vi "eventos.vi"() -> ()   [LabVIEW 2019]
uses:
  <vilib>/event_ctls.llb/eventvkey.ctl
panel:
  in  "MOUSE":bool
  out "ScanCode":i16
  out "PlatMods":T1
  out "VKey":T2
  out "Char":i16
  out "NewVal":bool
  out "OldVal":bool
  in  "Boolean":bool
  out "cuenta":i32
  in  "stop":bool
  in  "OK Button":bool
  out "iteraciones 1":i32
  out "LED 2":bool
  out "LED 1":bool
  # "EVENTO\nTECLADO"
  # "EVENTO\nCHANGE VALUE"
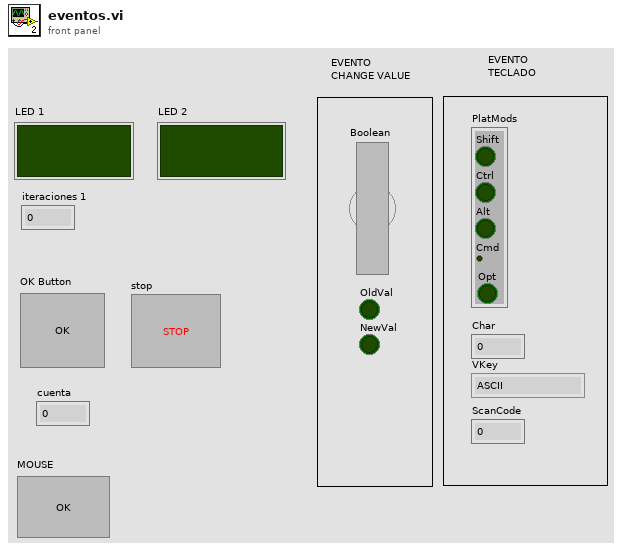
[diagram p1: front panel]
types:
  T1 = cluster{"Shift":bool, "Ctrl":bool, "Alt":bool, "Cmd":bool, "Opt":bool}
  T2 = typedef "eventvkey.ctl" = enum16{"ASCII", "Enter", "Return", "Shift", "Ctrl", "Alt", "Cmd", "Opt", "Caps", "NumLock", "Clear", "Break", "Up", "Down", "Left", "Right", "Insert", "Delete", "Home", "End", "PageUp", "PageDown", "Escape", "Help", "Pause", "ScrollLock", "F1", "F2", "F3", "F4", "F5", "F6", "F7", "F8", "F9", "F10", "F11", "F12", "F13", "F14", "F15", "F16", "F17", "F18", "F19", "F20", "F21", "F22", "F23", "F24", "Play", "VolumeUp", "VolumeDown", "Mute", "Two Byte Char"}
  T3 = typedef "LVPositionTypeDef.ctl" = cluster{"Left":i32, "Top":i32}
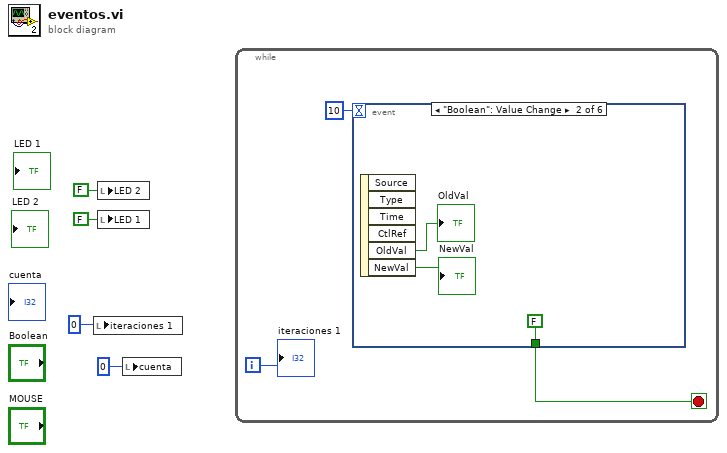
[diagram p0: block diagram]
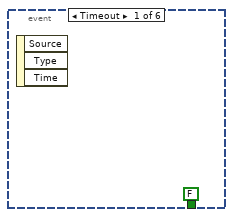
[diagram p2: hidden frame]
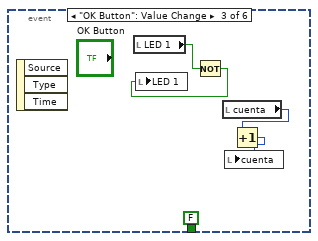
[diagram p3: hidden frame]
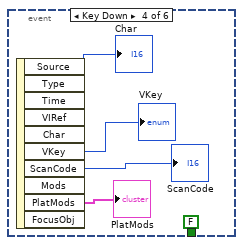
[diagram p4: hidden frame]
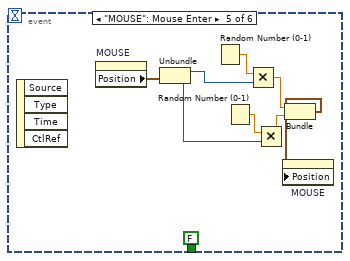
[diagram p5: hidden frame]
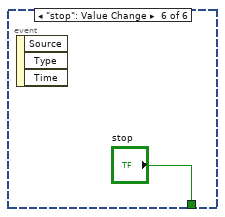
[diagram p6: hidden frame]
diagram:
  n1 = local write "iteraciones 1"(0 ("iteraciones 1")) -> ()
  n2 = local write "LED 2"(FALSE ("LED 2")) -> ()
  n3 = local write "LED 1"(FALSE ("LED 1")) -> ()
  n4 = local write "cuenta"(0 ("iteraciones 2")) -> ()
  n5 = while {
    i -> [w7]
    stop <- w6 stop-if-true
    n6 = event shown="[1] \"Boolean\": Value Change" {
      selector: _ -> [_ _ _ _ _ _]
      dyn-events: _ -> [_ _ _ _ _ _]
      timeout: 10 -> [_ _ _ _ _ _]
      tunnel: [FALSE ("stop") FALSE ("stop") FALSE ("stop") FALSE ("stop") FALSE ("stop") "stop"] -> w6
      event Timeout {
        n7 = event-data() -> ()  [unwired: 1 in, 3 out]
      }
      event "Boolean": Value Change {
        n8 = event-data() -> ("OldVal"=→"OldVal":bool, "NewVal"=→"NewVal":bool)  [unwired: 1 in, 4 out]
      }
      event "OK Button": Value Change {
        n9 = event-data() -> ()  [unwired: 1 in, 3 out]
        n10 = local read "LED 1"() -> (w16:bool)
        n11 = Not(x=w16) -> (.not. x?=w15:bool)
        n12 = local write "LED 1"(w15) -> ()
        n13 = local read "cuenta"() -> (w14:i32)
        n14 = Increment(x=w14) -> (x+1=w13:i32)
        n15 = local write "cuenta"(w13) -> ()
      }
      event Key Down {
        n16 = event-data() -> ("Char"=→"Char":i16, "VKey"=→"VKey":T2, "ScanCode"=→"ScanCode":i16, "PlatMods"=→"PlatMods":T1)  [unwired: 1 in, 6 out]
      }
      event "MOUSE": Mouse Enter {
        n17 = event-data() -> ()  [unwired: 1 in, 4 out]
        n18 = property on="MOUSE" class="Bool"() -> ("Position"=w30:T3)  [unwired: 2 in, 2 out]
        n19 = Unbundle(w30) -> ("Left"=w28:i32, "Top"=w26:i32)
        n20 = Random Number (0-1)() -> (number: 0 to 1=w29:dbl)
        n21 = Random Number (0-1)() -> (number: 0 to 1=w27:dbl)
        n22 = Multiply(x=w29, y=w28) -> (x*y=w25:dbl)
        n23 = Multiply(x=w27, y=w26) -> (x*y=w24:dbl)
        n24 = Bundle(w25, w24) -> (w23:cluster{dbl, dbl})  [unwired: 1 in]
        n25 = property on="MOUSE" class="Bool"("Position"=w23) -> ()  [unwired: 2 in, 2 out]
      }
      event "stop": Value Change {
        n26 = event-data() -> ()  [unwired: 1 in, 3 out]
      }
    }
    "iteraciones 1" <- w7
  }
